vi "Main__V2.vi"() -> (11 "Current Servo Status":cluster{"mode":string, "position":dbl})   [LabVIEW 2024]
panel:
  in  "New Servo Status":cluster{"mode":string, "position":dbl}
  in  "Set new status":bool
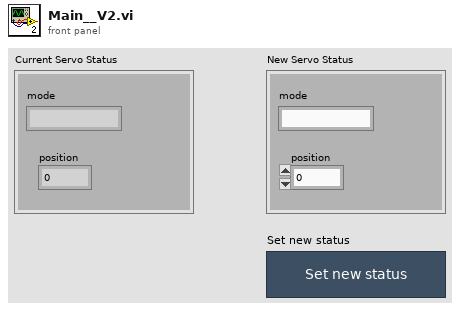
[diagram p1: front panel]
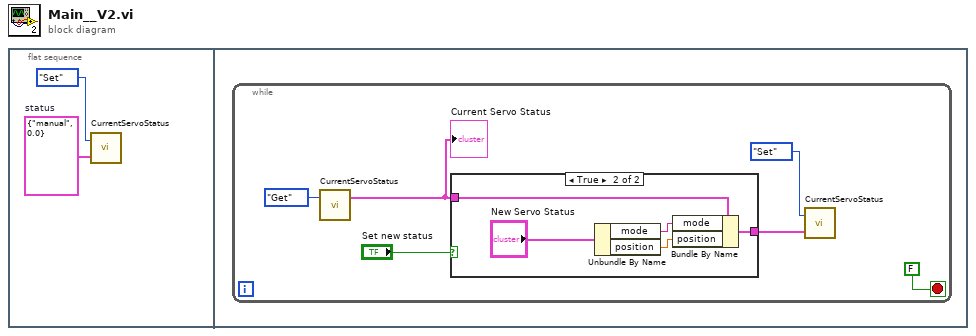
[diagram p0: block diagram]
diagram:
  n1 = flat-sequence {
    frame #0 {
      w1 = cluster{"mode":string, "position":dbl} {"mode"="manual", "position"=0.0}  # status
      n2 = call "CurrentServoStatus.vi"("New Servo Status"=w1, "Operation"=enum16{"Get", "Set", ""}."Set") -> ()  [unwired: 1 in, 1 out]
    }
    frame #1 {
      n3 = while {
        stop <- FALSE stop-if-true
        n4 = call "CurrentServoStatus.vi"("Operation"=enum16{"Get", "Set", ""}."Get") -> ("Current Servo Status"=w5:cluster{"mode":string, "position":dbl})  [unwired: 2 in]
        "Current Servo Status" <- w5
        n5 = case shown="True" "Set new status" {
          tunnel: w5 -> [w9 w10]
          tunnel: [w9 w11] -> w3
          frame False {
          }
          frame True {
            n6 = Unbundle By Name("New Servo Status") -> ("mode"=w12:string, "position"=w13:dbl)
            n7 = Bundle By Name(cluster=w10, "mode"=w12, "position"=w13) -> (w11:cluster{"mode":string, "position":dbl})
          }
        }
        n8 = call "CurrentServoStatus.vi"("New Servo Status"=w3, "Operation"=enum16{"Get", "Set", ""}."Set") -> ()  [unwired: 1 in, 1 out]
      }
    }
  }
